vi "Klinger OriginSearch.vi"(0 "Axe":u8(ring) items=["W", "X", "Y", "Z"], 1 "UnitDem":u8(ring)=2 caption="Unités\nDemandées" items=["Pas", "mm", "ps"], 5 "Moving Ref":refnum<vi>, 9 "Position Ref":refnum<vi>, 11 "error in":errorcluster, 12 "Set as Zero":bool) -> (2 "Pos Init":dbl caption="Position Initiale", 3 "Moving":bool caption="Déplacement\nen cours", 4 "PLimit":bool caption="Limite +", 6 "NLimit":bool caption="Limite -", 10 "Position":dbl format="%#.1f", 14 "Indcomm":string caption="Indicateur de commande", 15 "error out":errorcluster)   [LabVIEW 2010]
doc: "Ce VI envoie une commande de Mise à 0 au controlleur Klinger MC4. \n\nAxe : Sélectionner l'axe sur lequel effectuer la mise à zéro\n\nMoving Ref : Connecter une référence permet l'actualisation d'un afficheur de déplacement en cours en temp réelle\n\nPosition Ref: Connecter une référence permet l'actualisation d'un afficheur de position actuelle en temp réelle\n\nLimite + : Indique l'atteinte de l'interrupeur de fin de course positif\n\nLimite - : Indique l'atteinte de l'interrupeur de fin de course négatif\n\nPosition: Indique la position finale"
panel:
  out "Message D'erreur":string
  out "Erreur":bool
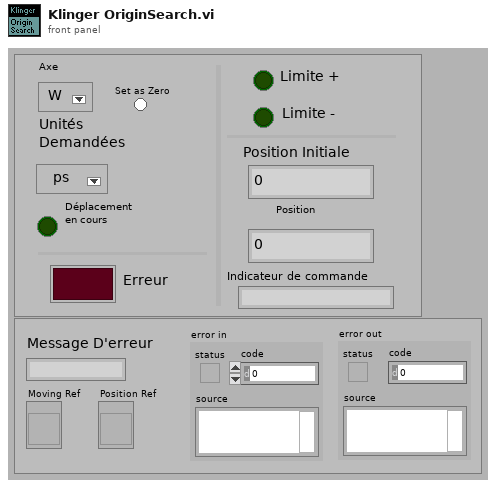
[diagram p1: front panel]
types:
  T1 = enum16{"Dem Pos Init", "Lire Pos Init", "Envoie Comm", "Dem Statut", "Lire Statut", "Attend RQS", "Erreur GPIB", "Dépl incomp", "Dépl comp"}
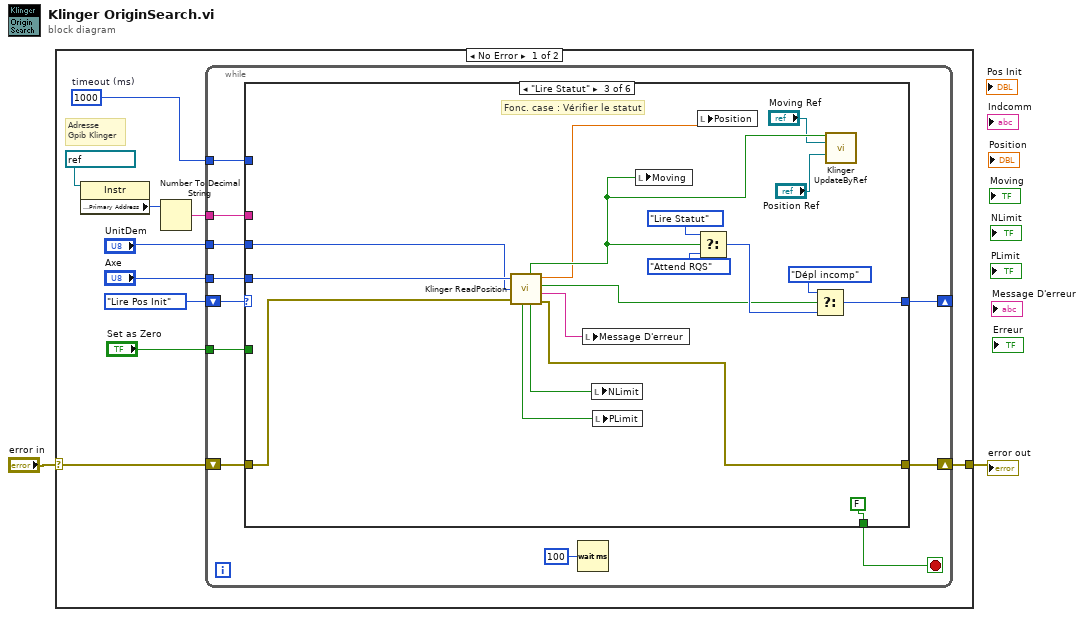
[diagram p0: block diagram]
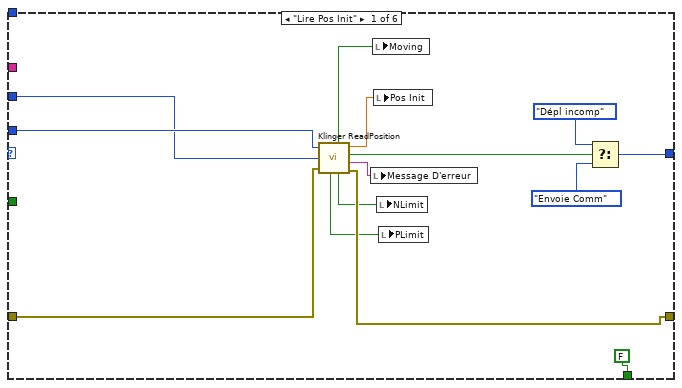
[diagram p2: hidden frame]
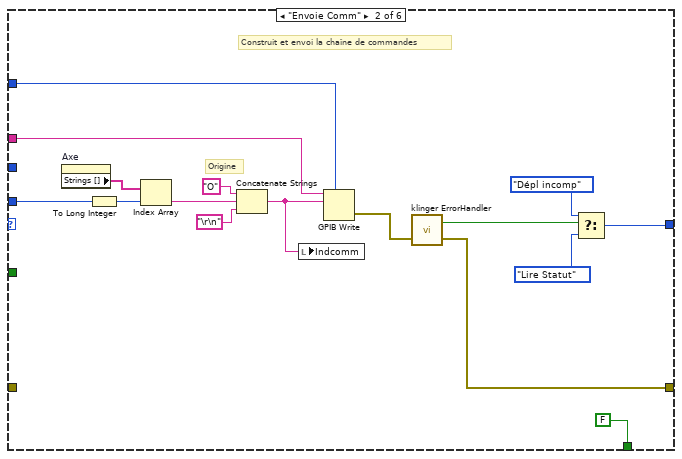
[diagram p3: hidden frame]
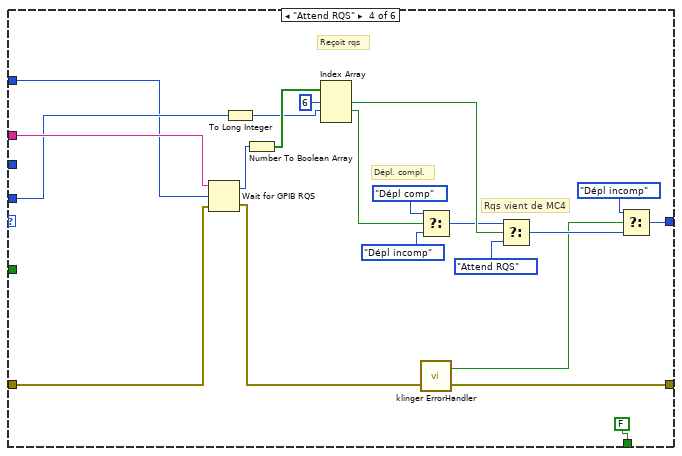
[diagram p4: hidden frame]
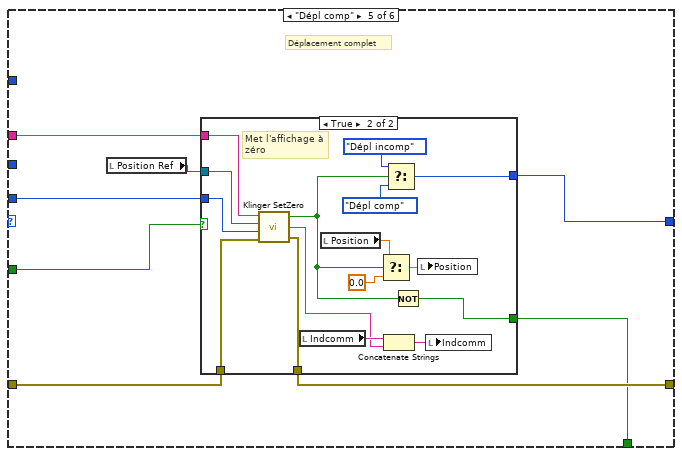
[diagram p5: hidden frame]
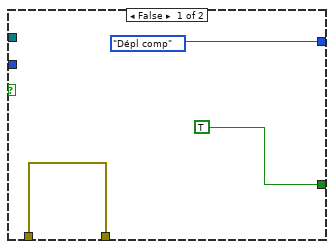
[diagram p6: hidden frame]
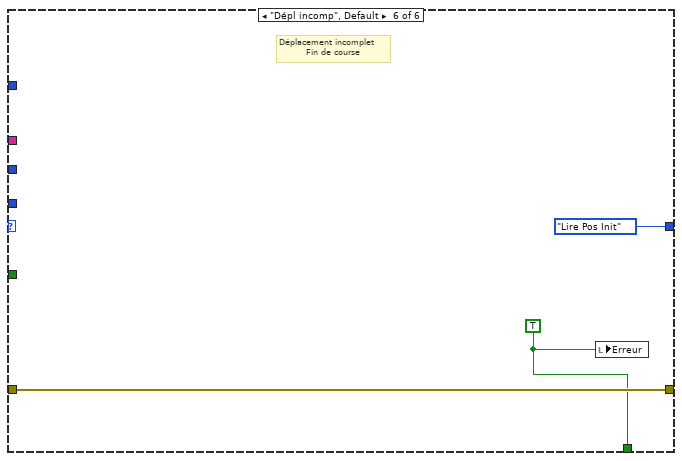
[diagram p7: hidden frame]
diagram:
  n1 = case shown="No Error" "error in" {
    selector: "error in" -> [w9 w123]
    tunnel: [w11 w123] -> w2
    frame No Error {
      w10 = 1000  # timeout (ms)
      # "Adresse \nGpib Klinger"
      n2 = property class="Instr"(reference=refnum<visa-resource-name> "KLINGER") -> ("GPIB Settings:Primary Address"=w6:u16)  [unwired: 1 in, 2 out]
      n3 = Number To Decimal String(number=w6) -> (decimal integer string=w4:string)  [unwired: 1 in]
      n4 = while {
        shift-right: [w22] -> w11
        shift-left: w9 -> [w21]
        tunnel: "Axe" -> [w20]
        tunnel: w4 -> [w19]
        tunnel: w10 -> [w18]
        shift-right: [w15] -> _
        shift-left: T1."Lire Pos Init" ("f") -> [w16]
        tunnel: "Set as Zero" -> [w14]
        tunnel: "UnitDem" -> [w13]
        stop <- w23 stop-if-true
        n5 = case shown="\"Lire Statut\"" w16 {
          tunnel: [FALSE FALSE FALSE FALSE w95 w120] -> w23
          tunnel: [w33 w39 w64 w73 w97 w121] -> w22
          tunnel: w21 -> [w31 _ w65 w92 w98 w121]
          tunnel: w20 -> [w30 w49 w62 w90 w99 _]
          tunnel: w19 -> [_ w47 _ w91 w93 _]
          tunnel: w18 -> [_ w46 _ w81 _ _]
          tunnel: [w34 w43 w68 w76 w96 T1."Lire Pos Init" ("f")] -> w15
          tunnel: w14 -> [_ _ _ _ w100 _]
          tunnel: w13 -> [w24 _ w55 _ _ _]
          frame "Lire Pos Init" {
            n6 = call <userlib>:"Klinger ReadPosition.vi"("Axe"=w30, "UnitDem"=w24, "error in"=w31) -> ("PLimit"=w26:bool, "Moving"=w28:bool, "Position"=w29:dbl, "Statut"=w32:bool, "NLimit"=w27:bool, "Cont Error"=w25:string, "error out"=w33:errorcluster)  [unwired: 1 in]
            n7 = local write "Message D'erreur"(w25) -> ()
            n8 = local write "Moving"(w28) -> ()
            n9 = local write "Pos Init"(w29) -> ()
            n10 = local write "NLimit"(w27) -> ()
            n11 = local write "PLimit"(w26) -> ()
            n12 = Select(t=T1."Dépl incomp", s=w32, f=T1."Envoie Comm") -> (s? t:f=w34:T1)
          }
          frame "Envoie Comm" {
            # "Origine"
            # "Construit et envoi la chaîne de commandes"
            n13 = property on="Axe" class="Ring (strict)"() -> ("Strings []"=w53:string[])  [unwired: 2 in, 2 out]
            n14 = To Long Integer(number=w49) -> (32bit integer=w48:i32)
            n15 = Index Array(array=w53, index=w48) -> (element=w52:string)
            n16 = Concatenate Strings("O", w52, "\r\n") -> (w40:string)
            n17 = local write "Indcomm"(w40) -> ()
            n18 = GPIB Write(0:w47, 1:w40, 4:w46) -> (6:w50:errorcluster)  [unwired: 2 in, 1 out]
            n19 = call <userlib>:"klinger ErrorHandler.vi"("error in (no error)"=w50) -> ("error out"=w39:errorcluster, "Erreur"=w38:bool)  [unwired: 1 in]
            n20 = Select(t=T1."Dépl incomp", s=w38, f=T1."Lire Statut") -> (s? t:f=w43:T1)
          }
          frame "Lire Statut" {
            # "Fonc. case : Vérifier le statut"
            n21 = call <userlib>:"Klinger ReadPosition.vi"("Axe"=w62, "UnitDem"=w55, "error in"=w65) -> ("PLimit"=w59:bool, "Moving"=w61:bool, "Position"=w54:dbl, "Statut"=w63:bool, "NLimit"=w60:bool, "Cont Error"=w58:string, "error out"=w64:errorcluster)  [unwired: 1 in]
            n22 = local write "Message D'erreur"(w58) -> ()
            n23 = local write "NLimit"(w60) -> ()
            n24 = local write "PLimit"(w59) -> ()
            n25 = local write "Moving"(w61) -> ()
            n26 = local write "Position"(w54) -> ()
            n27 = Select(t=T1."Lire Statut", s=w61, f=T1."Attend RQS") -> (s? t:f=w66:T1)
            n28 = Select(t=T1."Dépl incomp", s=w63, f=w66) -> (s? t:f=w68:T1)
            n29 = call <userlib>:"Klinger UpdateByRef.vi"("Moving?"=w61, "Moving Ref"="Moving Ref", "Position Ref"="Position Ref") -> ()  [unwired: 12 in, 1 out]
          }
          frame "Attend RQS" {
            # "Dépl. compl."
            # "Rqs vient de MC4"
            # "Reçoit rqs"
            n30 = Wait for GPIB RQS(2:w92, 3:w81, 4:w91) -> (0:w80:errorcluster, 1:w88:i16)
            n31 = To Long Integer(number=w90) -> (32bit integer=w84:i32)
            n32 = Number To Boolean Array(number=w88) -> (Boolean array=w89:bool[])
            n33 = Index Array(array=w89, index #1=6 ("index"), index #2=w84) -> (element #1=w86:bool, element #2=w83:bool)  [unwired: 1 in, 1 out]
            n34 = Select(t=T1."Dépl comp", s=w83, f=T1."Dépl incomp") -> (s? t:f=w82:T1)
            n35 = call <userlib>:"klinger ErrorHandler.vi"("error in (no error)"=w80) -> ("error out"=w73:errorcluster, "Erreur"=w72:bool)  [unwired: 1 in]
            n36 = Select(t=w82, s=w86, f=T1."Attend RQS") -> (s? t:f=w75:T1)
            n37 = Select(t=T1."Dépl incomp", s=w72, f=w75) -> (s? t:f=w76:T1)
          }
          frame "Dépl comp" {
            # "Déplacement complet"
            n38 = local read "Position Ref"() -> (w94:refnum<vi>)
            n39 = case shown="True" w100 {
              tunnel: w99 -> [_ w113]
              tunnel: w98 -> [w103 w114]
              tunnel: [w103 w115] -> w97
              tunnel: [T1."Dépl comp" w117] -> w96
              tunnel: [TRUE ("Stop") w116] -> w95
              tunnel: w94 -> [_ w105]
              tunnel: w93 -> [_ w104]
              frame False {
              }
              frame True {
                # "Met l'affichage à \nzéro"
                n40 = call <userlib>:"Klinger SetZero.vi"("Address GPIB"=w104, "Position Ref"=w105, "Axe"=w113, "error in"=w114) -> ("Statut"=w112:bool, "Ind Comm"=w106:string, "error out"=w115:errorcluster)  [unwired: 1 in]
                n41 = local read "Indcomm"() -> (w108:string)
                n42 = local read "Position"() -> (w110:dbl)
                n43 = Select(t=w110, s=w112, f=0.0) -> (s? t:f=w111:dbl)
                n44 = Concatenate Strings(w108, w106) -> (w107:string)
                n45 = Select(t=T1."Dépl incomp", s=w112, f=T1."Dépl comp") -> (s? t:f=w117:T1)
                n46 = Not(x=w112) -> (.not. x?=w116:bool)
                n47 = local write "Position"(w111) -> ()
                n48 = local write "Indcomm"(w107) -> ()
              }
            }
          }
          frame "Dépl incomp", Default {
            w120 = TRUE ("Stop")
            # "Déplacement incomplet\n         Fin de course"
            n49 = local write "Erreur"(w120) -> ()
          }
        }
        n50 = Wait (ms)(milliseconds to wait=u32 100) -> ()  [unwired: 1 out]
      }
    }
    frame Error {
    }
  }
  "error out" <- w2
